vi "State Machine Logging - ON or OFF.vi"(0 "reference in":refnum<class "Generic Utilities.lvclass">, 5 "error in (no error)":errorcluster, 7 "State Machine Logging?":bool) -> (14 "reference out":refnum<class "Generic Utilities.lvclass">, 19 "error out":errorcluster)   [LabVIEW 2022 SP3, in "Generic Utilities.lvclass"]
uses:
  Generic Utilities.lvclass
  <vilib>/Utility/sysdir.llb/System Directory Type.ctl
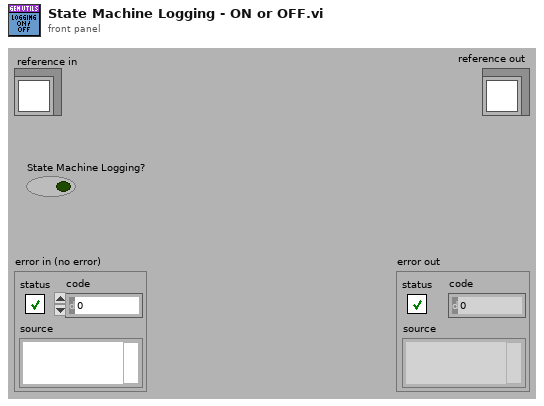
[diagram p1: front panel]
types:
  T1 = typedef "Generic Utilities.lvclass/ObjectAttributesRef.ctl" = refnum<data-value>
  T2 = typedef "Generic Utilities.lvclass/ObjectAttributes.ctl" = cluster{"GUI Parameters":T3, "State Machine Control":cluster{"Timeout":i32, "State Queue":string[], "State History":string[], "State History Length":i32}, "Logging File Path":path, "OBJ not a refnum?":bool, "Timer Start":timestamp, "FP Refnums":T4}
  T3 = typedef "Generic Utilities.lvclass/GUI Parameters.ctl" = cluster{"Application Name":string, "GUI VI Ref":refnum<vi>, "Close Panel?":bool, "Message Window ref":refnum<vi>, "Version #":string}
  T4 = typedef "Generic Utilities.lvclass/FP Refnums.ctl" = cluster{"Panel refnum":refnum<vi>, "Control Labels":string[], "Refnums":refnum<vi>[]}
  T5 = typedef "System Directory Type.ctl" = i32
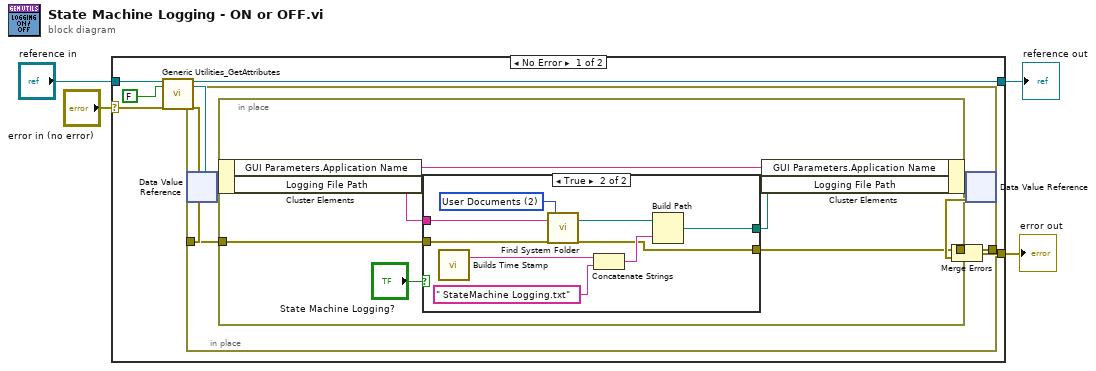
[diagram p0: block diagram]
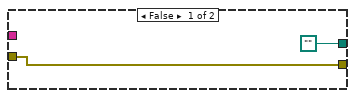
[diagram p2: hidden frame]
diagram:
  n1 = case shown="No Error" "error in (no error)" {
    selector: "error in (no error)" -> [w8 w35]
    tunnel: [w13 w35] -> w3
    tunnel: [w7 w34] -> w1
    tunnel: "reference in" -> [w10 w34]
    frame No Error {
      n2 = call "Generic Utilities_GetAttributes.vi"("reference in"=w10, "return data? (T)"=FALSE, "error in (no error)"=w8) -> ("reference out"=w7:refnum<class "Generic Utilities.lvclass">, "attributes ref"=w6:T1, "error out"=w5:errorcluster)  [unwired: 13 in, 1 out]
      n3 = in-place {
        in-place-border: [w14] -> w11
        in-place-border: w5 -> [w15]
        n4 = in-place-dvr #1(w6) -> (w16:T2)  [unwired: 1 out]
        n5 = in-place {
          in-place-border: w15 -> [w20]
          in-place-border: [w18] -> w14
          n6 = in-place-cluster #2(w16) -> ("GUI Parameters.Application Name"=w21:string)  [unwired: 1 out]
          n7 = case shown="True" "State Machine Logging?" {
            tunnel: w21 -> [_ w32]
            tunnel: w20 -> [w23 w31]
            tunnel: [path "" w26] -> w19
            tunnel: [w23 w25] -> w18
            frame False {
            }
            frame True {
              w33 = T5 2 items=["User Home"=0, "User Desktop"=1, "User Documents"=2, "User Application Data"=3, "User Preferences"=4, "User Temporary"=5, "Public Documents"=6, "Public Application Data"=7, "Public Preferences"=8, "Public Cache"=13, "System Core Libraries"=9, "System Installed Libraries"=10, "Application Files"=11, "Boot Volume Root"=12] ("system directory type")
              n8 = call "Builds Time Stamp.vi"() -> ("TimeStamp"=w30:string)  [unwired: 19 in]
              n9 = call "Find System Folder.vi"("Application Name"=w32, "error in (no error)"=w31, "system directory type"=w33) -> ("System Folder"=w28:path, "error out"=w25:errorcluster)  [unwired: 15 in]
              n10 = Concatenate Strings(w30, " StateMachine Logging.txt" ("string")) -> (w27:string)
              n11 = Build Path(base path=w28, name or relative path=w27) -> (appended path=w26:path)
            }
          }
          n12 = in-place-cluster #2("GUI Parameters.Application Name"=w21, "Logging File Path"=w19) -> (w17:T2)
        }
        n13 = in-place-dvr #1(w17) -> (w12:errorcluster)  [unwired: 1 out]
      }
      n14 = Merge Errors(w11, w12) -> (w13:errorcluster)
    }
    frame Error {
    }
  }
  "error out" <- w3
  "reference out" <- w1
